vi "cRIO HOST.vi"(8 "error in":errorcluster, 10 "resource name":T1 caption="RIO Device", 11 "MeasSet":T2={"Data Rate 9775"=20.0, "Data Rate 9215"=20.0, "Samples RMS 9215"=10000, "Samples RMS 9775"=10000}) -> (0 "Host error out":errorcluster, 1 "Start time":timestamp=timestamp(3682932872.9709415 s since 1904-01-01), 2 "data 9775x2":dbl[](array[numeric])=[-0.002410888671875, 3.0517578125e-05, -10.432037353515625, -10.390777587890625, -0.002410888671875, 3.0517578125e-05, -10.432037353515625, -10.390777587890625, -0.002105712890625, 0.00067138671875, -10.432037353515625, -10.390777587890625, -0.002410888671875, -0.000274658203125, -10.432037353515625, -10.390777587890625, -0.002105712890625, 3.0517578125e-05, -10.432037353515625, -10.390777587890625, -0.002410888671875, 3.0517578125e-05, -10.432037353515625, -10.390777587890625, -0.002410888671875, 0.0003662109375, -10.432037353515625, -10.390777587890625, -0.002105712890625, -0.000274658203125, -10.432037353515625, -10.390777587890625, -0.0030517578125, 0.00067138671875, -10.432037353515625, -10.390777587890625, -0.0030517578125, -0.000274658203125, -10.432037353515625, -10.390777587890625, -0.002410888671875, 3.0517578125e-05, -10.432037353515625, -10.390777587890625, -0.00274658203125, -0.000274658203125, -10.432037353515625, -10.390777587890625, -0.0030517578125, -0.000274658203125, -10.432037353515625, -10.390777587890625, -0.002410888671875, 0.0003662109375, -10.432037353515625, -10.390777587890625, -0.003387451171875, 3.0517578125e-05, -10.432037353515625, -10.390777587890625, -0.00274658203125, -0.000274658203125, -10.432037353515625, -10.390777587890625, -0.00274658203125, 3.0517578125e-05, -10.432037353515625, -10.390777587890625, -0.002410888671875, -0.000274658203125, -10.432037353515625, -10.390777587890625, -0.002410888671875, 0.0003662109375, -10.432037353515625, -10.390777587890625, -0.00274658203125, 0.0003662109375, -10.432037353515625, -10.390777587890625, -0.002410888671875, 3.0517578125e-05, -10.432037353515625, -10.390777587890625, -0.002410888671875, 3.0517578125e-05, -10.432037353515625, -10.390777587890625, -0.00274658203125, -0.000274658203125, -10.432037353515625, -10.390777587890625, -0.003692626953125, 3.0517578125e-05, -10.432037353515625, -10.390777587890625, -0.002410888671875, 3.0517578125e-05, -10.432037353515625, -10.390777587890625, -0.0030517578125, 3.0517578125e-05, -10.432037353515625, -10.390777587890625, -0.003387451171875, 0.0003662109375, -10.432037353515625, -10.390777587890625, -0.003387451171875, 0.0003662109375, -10.432037353515625, -10.390777587890625, -0.0030517578125, 0.00067138671875, -10.432037353515625, -10.390777587890625, -0.0030517578125, 3.0517578125e-05, -10.432037353515625, -10.390777587890625, -0.0030517578125, 0.0003662109375, -10.432037353515625, -10.390777587890625, -0.0030517578125, 3.0517578125e-05, -10.432037353515625, -10.390777587890625], 3 "data 9215":dbl[](array[numeric])=[0.00146484375, 0.00048828125, -0.0029296875, 0.001953125, 0.0009765625, 0.002197265625, 0.0048828125, -0.000732421875, -0.002685546875, -0.002197265625, -0.00146484375, 0.004638671875, -0.000244140625, -0.000732421875, 0.002197265625, -0.000732421875, -0.002685546875, -0.0009765625, 0.001220703125, -0.0009765625, 0.00244140625, -0.006103515625, 0.0048828125, 0.001953125, 0.0, -0.002197265625, 0.0, 0.001953125, 0.003662109375, -0.00341796875, 0.010498046875, -0.000732421875, -0.002685546875, -0.005126953125, 0.0, 0.003173828125, -0.001708984375, 0.000732421875, 0.002197265625, -0.000732421875, -0.004150390625, -0.002197265625, -0.0068359375, 0.003173828125, 0.00244140625, -0.000732421875, 0.00341796875, 0.00341796875, 0.007080078125, -0.0009765625, 0.001220703125, 0.00048828125, -0.00439453125, -0.000732421875, 0.002197265625, 0.00341796875, 0.0, -0.002197265625, -0.00146484375, 0.003173828125, -0.00439453125, -0.00341796875, 0.000732421875, 0.001953125, -0.002685546875, -0.002197265625, 0.0068359375, 0.001953125, -0.003173828125, -0.000732421875, 0.002197265625, 0.001953125, 0.0029296875, 0.00048828125, 0.002685546875, -0.0009765625, -0.001708984375, -0.000732421875, 0.002197265625, -0.000732421875, 0.0, -0.002197265625, 0.002685546875, -0.002197265625, -0.000244140625, 0.000732421875, 0.007568359375, 0.001953125, -0.00537109375, -0.0009765625, -0.0029296875, 0.001953125, 0.0009765625, 0.002197265625, 0.00634765625, 0.00341796875, -0.001220703125, 0.001953125, -0.00146484375, 0.00048828125, -0.000244140625, -0.004638671875, 0.00341796875, 0.0048828125, 0.0, -0.003662109375, 0.0, 0.001953125, 0.00244140625, 0.000732421875, 0.0048828125, 0.001953125, 0.00146484375, -0.002197265625, 0.002685546875, -0.002197265625, -0.000244140625, 0.000732421875, 0.00341796875, 0.000732421875, 0.00146484375, 0.001953125, -0.00146484375, 0.003173828125, -0.000244140625, -0.000732421875, 0.0048828125, 0.000732421875, 0.00146484375, -0.003662109375, 0.001220703125, 0.00048828125, -0.003173828125, -0.001953125, 0.00634765625, -0.002197265625, 0.004150390625, -0.002197265625, 0.002685546875, 0.001953125, -0.005859375, -0.000732421875, 0.0048828125, 0.00341796875, 0.00146484375, 0.00048828125, 0.0, 0.003173828125, 0.0009765625, 0.000732421875, 0.007568359375, 0.006103515625, -0.001220703125, -0.0009765625, 0.002685546875, 0.001953125, -0.00439453125, -0.00341796875, 0.007568359375, 0.001953125, 0.004150390625, -0.0078125, -0.00146484375, 0.00048828125, -0.00439453125, -0.004638671875, 0.0048828125, 0.00341796875, 0.0, -0.002197265625, -0.00146484375, 0.003173828125, -0.00439453125, -0.000732421875, 0.00634765625, 0.001953125, 0.0, -0.003662109375, 0.0, 0.004638671875, -0.000244140625, -0.004638671875, 0.009033203125, 0.000732421875, -0.002685546875, -0.005126953125, 0.0, 0.00048828125, -0.005859375, -0.001953125, 0.00341796875, -0.00341796875, 0.004150390625, -0.003662109375, 0.004150390625, -0.002197265625, -0.000244140625, -0.00341796875, 0.00341796875, -0.00341796875, 0.004150390625, -0.002197265625, -0.0029296875, -0.002197265625, 0.00244140625, -0.000732421875, 0.0048828125, -0.000732421875, 0.0029296875, 0.00048828125, 0.004150390625, 0.00048828125, 0.00244140625, 0.000732421875, 0.002197265625, -0.00341796875, -0.001220703125, 0.00048828125, 0.0, -0.0009765625, -0.001708984375, -0.000732421875, 0.0048828125, 0.000732421875, -0.001220703125, -0.0009765625, 0.0, 0.006103515625, -0.003173828125, -0.00341796875, 0.0048828125, 0.006103515625, -0.002685546875, -0.00634765625, 0.001220703125, -0.002197265625, -0.00439453125, 0.000732421875, 0.002197265625, 0.000732421875, 0.0, 0.00048828125, -0.00146484375, -0.003662109375, -0.000244140625, -0.000732421875, -0.000732421875, -0.002197265625, -0.001220703125, -0.0009765625, 0.0, -0.003662109375, -0.000244140625, 0.000732421875, -0.000732421875, 0.001953125, -0.001220703125, -0.002197265625, 0.0, 0.003173828125, 0.0009765625, -0.000732421875, -0.000732421875, 0.000732421875, -0.002685546875, -0.002197265625, 0.0, 0.00048828125, -0.001708984375, 0.002197265625, 0.00341796875, -0.0048828125, 0.0, -0.002197265625, 0.001220703125, 0.00048828125, -0.005859375, 0.000732421875, 0.0048828125, 0.001953125, -0.001220703125, -0.003662109375, 0.001220703125, 0.00048828125, -0.00439453125, 0.000732421875, 0.0048828125, -0.002197265625, -0.001220703125, 0.001953125, 0.004150390625, 0.001953125, -0.001708984375, 0.000732421875, 0.00634765625, 0.0048828125, -0.004150390625, -0.0009765625, 0.001220703125, -0.0009765625, 0.0009765625, -0.001953125, 0.002197265625, -0.002197265625, -0.002685546875, -0.002197265625, 0.0, 0.00732421875, 0.0009765625, -0.001953125, 0.0048828125, 0.000732421875, 0.00146484375, -0.003662109375, 0.002685546875, 0.003173828125, -0.00439453125, -0.004638671875, -0.001953125, 0.001953125, -0.004150390625, -0.005126953125, 0.004150390625, 0.00048828125, 0.003662109375, -0.00341796875, -0.001953125, 0.0048828125, -0.002685546875, -0.0009765625, 0.0, 0.003173828125, 0.0009765625, -0.000732421875, 0.00634765625, -0.000732421875, 0.00146484375, 0.001953125, 0.001220703125, 0.00048828125, 0.0009765625, -0.000732421875, 0.002197265625, 0.00341796875, -0.001220703125, -0.002197265625, 0.0, 0.00048828125, 0.0009765625, -0.001953125, 0.002197265625, -0.000732421875, 0.00146484375, -0.0009765625, 0.002685546875, 0.003173828125, 0.00244140625, -0.000732421875, 0.00634765625, 0.001953125, 0.0, -0.002197265625, -0.0029296875, 0.003173828125, -0.000244140625, -0.001953125, -0.001953125, 0.001953125, -0.001220703125, 0.003173828125, -0.0029296875, 0.003173828125, -0.00439453125, -0.001953125, 0.00634765625, -0.002197265625, -0.001220703125, 0.001953125, -0.0029296875, 0.00048828125, 0.003662109375, 0.000732421875, 0.002197265625, 0.001953125, 0.0, -0.0009765625, -0.00146484375, 0.003173828125, -0.00439453125, -0.001953125, 0.0048828125, 0.000732421875, 0.00146484375, -0.0009765625, 0.002685546875, 0.00048828125, 0.003662109375, -0.000732421875, -0.000732421875, -0.000732421875, 0.0, 0.003173828125, -0.004150390625, 0.003173828125, 0.0009765625, 0.0048828125, 0.00341796875, 0.0048828125, -0.004150390625, 0.001953125, 0.002685546875, 0.001953125, 0.003662109375, 0.002197265625, 0.00634765625, -0.000732421875, -0.001220703125, 0.001953125, 0.002685546875, 0.001953125, -0.001708984375, 0.00341796875, 0.009033203125, 0.000732421875, -0.001220703125, -0.002197265625, 0.0, 0.003173828125, 0.003662109375, 0.000732421875, 0.009033203125, -0.00634765625, 0.0029296875, -0.0009765625, -0.00146484375, -0.002197265625, 0.0009765625, -0.000732421875, 0.00634765625, 0.000732421875, -0.004150390625, -0.005126953125, 0.001220703125, 0.00048828125, 0.0009765625, 0.00341796875, 0.009033203125, -0.002197265625, 0.00146484375, 0.00048828125, 0.0, 0.003173828125, -0.000244140625, -0.004638671875, 0.0048828125, 0.000732421875, -0.00537109375, -0.002197265625, -0.004150390625, -0.0009765625, -0.001708984375, -0.000732421875, 0.00634765625, -0.002197265625, 0.0029296875, 0.00048828125, -0.0029296875, 0.00048828125, -0.000244140625, 0.000732421875, 0.00634765625, 0.0048828125, -0.001220703125, -0.003662109375, 0.001220703125, -0.002197265625, -0.005859375, -0.00341796875, 0.00341796875, 0.001953125, -0.002685546875, -0.0009765625, 0.0, -0.002197265625, -0.005859375, -0.000732421875, 0.00634765625, 0.001953125, 0.004150390625, -0.003662109375, 0.001220703125, 0.00048828125, -0.001708984375, 0.000732421875, 0.002197265625, 0.000732421875, 0.00146484375, -0.003662109375, -0.00146484375, -0.002197265625, -0.003173828125, -0.00341796875, 0.00341796875, 0.00341796875, 0.0, 0.001953125, 0.004150390625, 0.006103515625, -0.001708984375, 0.00341796875, 0.002197265625, -0.000732421875, 0.004150390625, -0.0009765625, 0.008056640625, 0.003173828125, -0.000244140625, -0.001953125, 0.007568359375, 0.00341796875, -0.004150390625, 0.003173828125, 0.002685546875, 0.003173828125, -0.001708984375, -0.000732421875, 0.0048828125, 0.001953125, -0.00537109375, -0.002197265625, -0.00146484375, -0.002197265625, 0.00244140625, -0.000732421875, 0.0048828125, 0.001953125, 0.00146484375, -0.0009765625, 0.004150390625, 0.003173828125, 0.0009765625, -0.004638671875, 0.000732421875, 0.001953125, 0.0, 0.001953125, 0.002685546875, 0.001953125, -0.000244140625, -0.00341796875, 0.0048828125, 0.000732421875, -0.001220703125, 0.003173828125, 0.0, 0.00048828125, -0.000244140625, 0.000732421875, 0.0048828125, 0.00341796875, 0.00146484375, 0.001953125, 0.002685546875, -0.0009765625, -0.000244140625, 0.000732421875, 0.002197265625, 0.00341796875, -0.001220703125, -0.003662109375, 0.001220703125, 0.00048828125, -0.000244140625, 0.000732421875, 0.00341796875, 0.00341796875, 0.0, -0.005126953125, 0.002685546875, 0.003173828125, -0.003173828125, 0.0048828125, 0.0048828125, 0.001953125, 0.0, -0.0009765625, 0.002685546875, 0.001953125, -0.00439453125, -0.000732421875, 0.00341796875, 0.0048828125, -0.001220703125, -0.0009765625, 0.004150390625, 0.001953125, -0.005859375, 0.000732421875, 0.0048828125, 0.000732421875, 0.007080078125, -0.002197265625, 0.004150390625, 0.001953125, -0.000244140625, -0.000732421875, 0.00341796875, 0.001953125, -0.002685546875, 0.003173828125, -0.0029296875, -0.002197265625, -0.001708984375, -0.004638671875, 0.00634765625, 0.001953125, -0.004150390625, -0.0009765625, 0.001220703125, 0.001953125, -0.00439453125, 0.00341796875, 0.00341796875, 0.00341796875, 0.00146484375, 0.003173828125, 0.0, 0.003173828125, -0.000244140625, -0.000732421875, 0.00634765625, -0.002197265625, 0.0, 0.001953125, 0.001220703125, 0.001953125, -0.00439453125, 0.00341796875, 0.000732421875, 0.001953125, 0.00146484375, 0.00048828125, 0.001220703125, 0.003173828125, -0.00732421875, 0.000732421875, 0.002197265625, -0.000732421875, -0.004150390625, 0.003173828125, -0.00146484375, 0.003173828125, -0.000244140625, -0.001953125, 0.00341796875, -0.000732421875, 0.007080078125, 0.003173828125, 0.004150390625, -0.002197265625, 0.0009765625, -0.000732421875, 0.0048828125, 0.001953125, -0.001220703125, -0.0009765625, -0.00146484375, 0.001953125, -0.00732421875, -0.000732421875, 0.0048828125, -0.000732421875, -0.004150390625, 0.001953125, 0.001220703125, 0.003173828125, -0.00732421875, 0.000732421875, 0.007568359375, -0.00341796875, 0.00146484375, -0.002197265625, 0.004150390625, -0.0009765625, -0.00439453125, -0.001953125, 0.0048828125, 0.000732421875, -0.00537109375, 0.00048828125, 0.001220703125, 0.00048828125, -0.00439453125, -0.00341796875, 0.0048828125, -0.000732421875, -0.002685546875, 0.00048828125, 0.0, 0.001953125, -0.001708984375, -0.000732421875, 0.0048828125, -0.000732421875, 0.0, -0.002197265625, 0.001220703125, -0.0009765625, -0.005859375, -0.000732421875, 0.000732421875, 0.00341796875, -0.002685546875, -0.0009765625, 0.0, -0.0009765625, 0.0009765625, -0.00341796875, 0.00634765625, 0.00341796875, -0.002685546875, -0.002197265625, 0.002685546875, 0.001953125, 0.0009765625, -0.001953125, 0.000732421875, -0.002197265625, 0.0029296875, 0.00048828125, -0.00146484375, 0.001953125, -0.00439453125, -0.00341796875, 0.007568359375, -0.000732421875, 0.0029296875, 0.001953125, 0.004150390625, 0.003173828125, -0.000244140625, -0.001953125, 0.00341796875, 0.000732421875, -0.00537109375, 0.00048828125, 0.0, 0.00048828125, -0.000244140625, -0.00341796875, -0.001953125, -0.002197265625, 0.0, -0.003662109375, -0.00146484375, -0.0009765625, -0.003173828125, -0.001953125, 0.0048828125, 0.000732421875, 0.00146484375, 0.00048828125, 0.0, 0.00048828125, 0.00244140625, -0.000732421875, 0.00341796875, 0.000732421875, -0.00537109375, -0.002197265625, -0.0029296875, 0.001953125, -0.003173828125, -0.000732421875, 0.0048828125, 0.000732421875, -0.002685546875, -0.002197265625, 0.001220703125, -0.002197265625, -0.000244140625, -0.001953125, 0.0048828125, -0.000732421875, -0.002685546875, 0.001953125, 0.0, 0.001953125, -0.000244140625, -0.001953125, 0.009033203125, 0.000732421875, -0.001220703125, 0.003173828125, 0.001220703125, -0.0009765625, -0.00732421875, -0.006103515625, 0.000732421875, -0.002197265625, -0.00537109375, -0.002197265625, -0.00146484375, -0.002197265625, -0.000244140625, -0.0087890625, 0.00341796875, 0.000732421875, -0.001220703125, 0.00048828125, 0.001220703125, -0.003662109375, -0.000244140625, -0.000732421875, 0.00341796875, 0.001953125, -0.002685546875, 0.003173828125, -0.004150390625, -0.0009765625, -0.001708984375, 0.00341796875, 0.000732421875, -0.000732421875, -0.002685546875, -0.0009765625, 0.002685546875, -0.002197265625, -0.001708984375, -0.001953125, 0.00341796875, 0.000732421875, -0.004150390625, -0.0009765625, -0.00146484375, -0.002197265625, 0.003662109375, -0.001953125, 0.0048828125, -0.00341796875, 0.00146484375, -0.003662109375, -0.00146484375, 0.00048828125, -0.000244140625, -0.000732421875, 0.007568359375, 0.00341796875, 0.0029296875, 0.001953125, -0.004150390625, -0.0009765625, -0.00439453125, 0.0048828125, 0.00341796875, -0.00341796875, -0.002685546875, 0.004638671875, 0.001220703125, 0.001953125, -0.003173828125, -0.000732421875, -0.000732421875, -0.00634765625, -0.004150390625, 0.001953125, 0.0, 0.003173828125, -0.000244140625, -0.000732421875, 0.000732421875, 0.001953125, 0.00146484375, -0.002197265625, 0.001220703125, 0.001953125, 0.0009765625, -0.001953125, 0.0048828125, -0.000732421875, -0.004150390625, -0.002197265625, 0.002685546875, -0.0009765625, -0.001708984375, 0.000732421875, 0.00341796875, 0.001953125, 0.00146484375, 0.001953125, 0.004150390625, -0.0009765625, 0.0009765625, -0.00341796875, 0.00341796875, -0.002197265625], 4 "Data FIFO Full":bool=TRUE, 6 "Data2 FIFO Full":bool=TRUE)   [LabVIEW 2019, in "DAQ_Engine.lvclass"]
uses:
  DAQ_Engine.lvclass
  Common/DataTypes/Measurement Config--cluster.ctl
  <vilib>/userdefined/High Color/nirio_resource_hc.ctl
  <vilib>/LabVIEW Targets/FPGA/cRIO/shared/nicrio_ModuleControls/nicrio_BasicConversionTime.ctl
  <vilib>/rvi/interface/RandomDataEmulation/nirviRandomDataOpen.vi
  <vilib>/rvi/interface/common/niFpgaCacheSessionInfoDynamic.vi
  <vilib>/Utility/error.llb/Error Cluster From Error Code.vi
  <vilib>/rvi/errors/niLvFpgaAdjustHostInterfaceError.vi
  <vilib>/FPGAPlugInAG/Dynamic/niLvFpga_Run_Dynamic.vi
  <vilib>/FPGAPlugInAG/Dynamic/niLvFpga_Close_Dynamic.vi
  <vilib>/rvi/interface/nirviOpenFPGA/nirviOpenFPGA.xnode
  FPGA/Acquisitions (FPGA).vi
  <vilib>/rvi/interface/nirviReadWriteControl/nirviReadWriteControl.xnode
  <vilib>/rvi/interface/nirviMethod/nirviMethod.xnode
  <vilib>/rvi/interface/nirviCloseFPGA/nirviCloseFPGA.xnode
  <vilib>/FPGAPlugInAG/Dynamic/niLvFpga_ReadFifo_Dynamic.vi
  <vilib>/rvi/errors/niLvFpgaMergeErrorWithErrorCode.vi
  <vilib>/rvi/interface/Simulation/niFpgaSimulationCallBeginRW.vi
  NiFpgaLv.dll
panel:
  out "Elements Remaining 2":u32=15488
  in  "stop":bool
  out "FPGA error out":errorcluster
  out "Elements Remaining":u32=3967
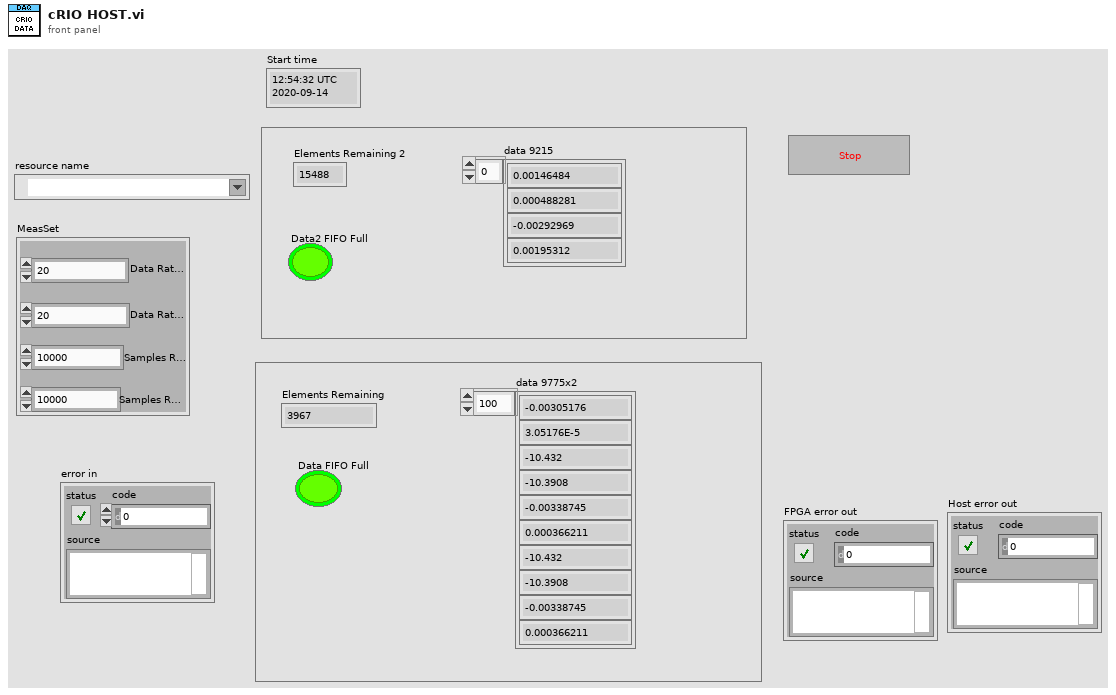
[diagram p1: front panel]
types:
  T1 = typedef "nirio_resource_hc.ctl" = tag
  T2 = typedef "Measurement Config--cluster.ctl" = cluster{"Data Rate 9775":dbl, "Data Rate 9215":dbl, "Samples RMS 9215":u32, "Samples RMS 9775":u32}
  T3 = typedef "nicrio_BasicConversionTime.ctl" = enum8{"High Speed", "High Resolution"}
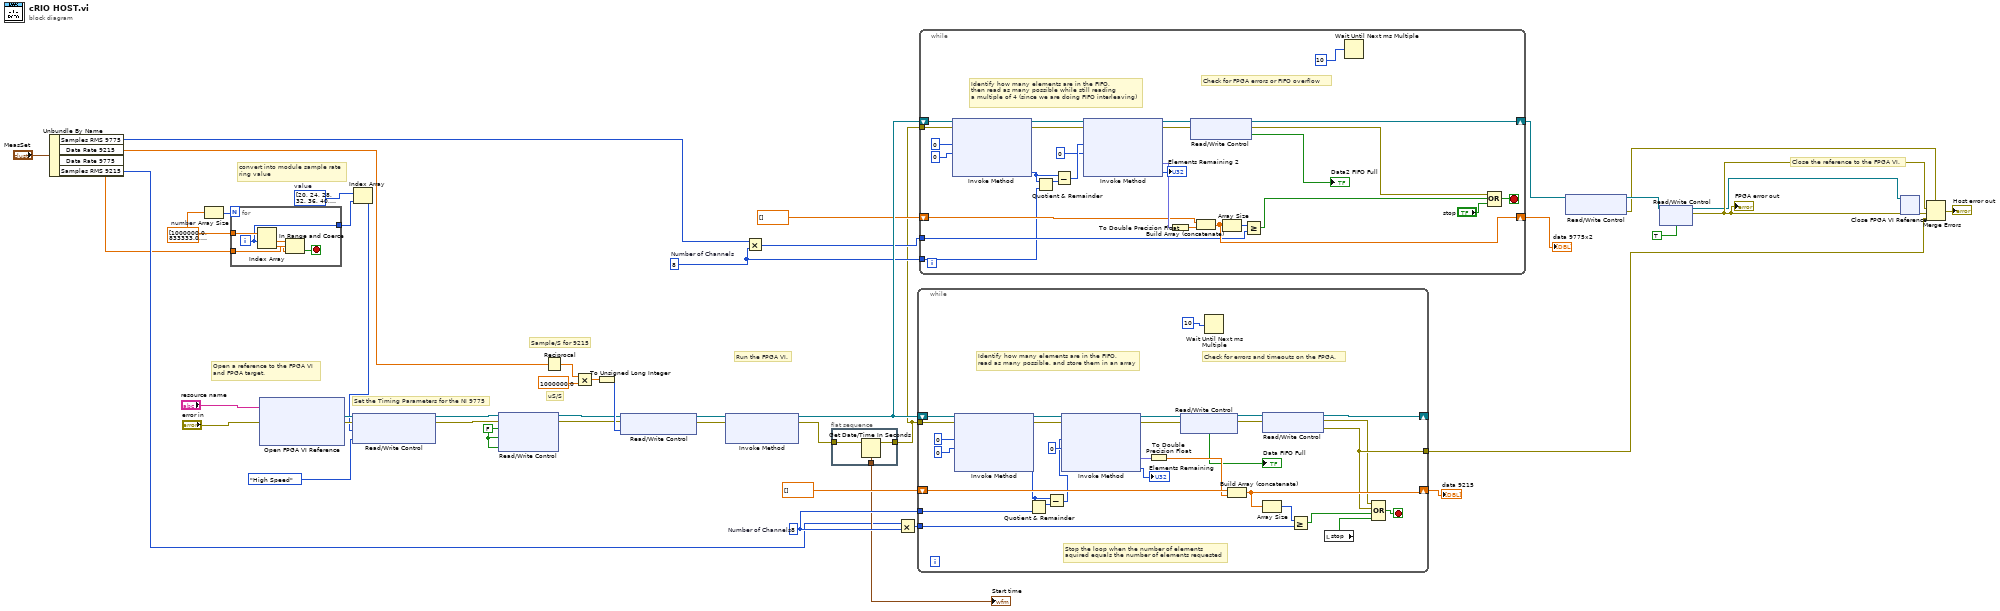
[diagram p0: block diagram]
diagram:
  w3 = u16[] [20, 24, 28, 32, 36, 40, 44, 48, 52, 56, 60, 64, 68, 72, 76, 80, 84, 88, 92, 96, 100, 104, 108, 112, 116, 120, 124, 128, 132, 136, 140, 144, 148, 152, 156, 160, 164, 168, 172, 176, 180, 184, 188, 192, 196, 200, 400, 600, 800, 1000, 1200, 1400, 1600, 1800, 2000, 2200, 2400, 2600, 2800, 3000, 3200, 3400, 3600, 4000, 4200, 4400, 4600, 4800, 5000, 5200, 5600, 6000, 6400, 6800, 7200, 7600, 8000, 8400, 8800, 9200, 9600, 10000, 10400, 10800, 11200, 11600, 12000, 12400, 12800, 13200, 13600, 14000, 14400, 14800, 15200, 15600, 16000, 16400, 16800, 17200, 17600, 18000, 18400, 18800, 19200, 19600, 20000, 20400, 20800, 21200, 21600, 22000, 22400, 22800, 23200, 23600, 24000, 24400, 24800, 25200, 25600, 28800, 32000, 35200, 38400, 44800, 51200, 57600, 64000]  # value
  w5 = dbl[] [1000000.0, 833333.0, 714286.0, 625000.0, 555556.0, 500000.0, 454545.0, 416667.0, 384615.0, 357143.0, 333333.0, 312500.0, 294118.0, 277778.0, 263158.0, 250000.0, 238095.0, 227273.0, 217391.0, 208333.0, 200000.0, 192308.0, 185185.0, 178571.0, 172414.0, 166667.0, 161290.0, 156250.0, 151515.0, 147059.0, 142857.0, 138889.0, 135135.0, 131579.0, 128205.0, 125000.0, 121951.0, 119048.0, 116279.0, 113636.0, 111111.0, 108696.0, 106383.0, 104167.0, 102041.0, 100000.0, 50000.0, 33333.0, 25000.0, 20000.0, 16667.0, 14286.0, 12500.0, 11111.0, 10000.0, 9091.0, 8333.0, 7692.0, 7143.0, 6667.0, 6250.0, 5882.0, 5556.0, 5000.0, 4762.0, 4545.0, 4348.0, 4167.0, 4000.0, 3846.0, 3571.0, 3333.0, 3125.0, 2941.0, 2778.0, 2632.0, 2500.0, 2381.0, 2273.0, 2174.0, 2083.0, 2000.0, 1923.0, 1852.0, 1786.0, 1724.0, 1667.0, 1613.0, 1563.0, 1515.0, 1471.0, 1429.0, 1389.0, 1351.0, 1316.0, 1282.0, 1250.0, 1220.0, 1190.0, 1163.0, 1136.0, 1111.0, 1087.0, 1064.0, 1042.0, 1020.0, 1000.0, 980.0, 962.0, 943.0, 926.0, 909.0, 893.0, 877.0, 862.0, 847.0, 833.0, 820.0, 806.0, 794.0, 781.0, 694.0, 625.0, 568.0, 521.0, 446.0, 391.0, 347.0, 313.0]  # number
  w18 = FALSE ("Data2 FIFO Full")
  w32 = u32 8  # Number of Channels
  w35 = u32 8  # Number of Channels
  # "convert into module sample rate\nring value"
  # "Sample/S for 9215"
  # "uS/S"
  # "Set the Timing Parameters for the NI 9775"
  # "Close the reference to the FPGA VI."
  # "Run the FPGA VI."
  # "Open a reference to the FPGA VI \nand FPGA target."
  n1 = Unbundle By Name("MeasSet") -> ("Samples RMS 9775"=w25:u32, "Data Rate 9215"=w11:dbl, "Data Rate 9775"=w6:dbl, "Samples RMS 9215"=w24:u32)
  n2 = Array Size(array=w5) -> (size(s)=w4:i32)
  n3 = for {
    N: w4 -> [_]
    tunnel: w5 -> [w53]
    tunnel: w6 -> [w51]
    tunnel: [w48] -> w2
    i -> [w48]
    stop <- w49 stop-if-true
    n4 = Index Array(array=w53, index #1=w48) -> (element #1=w52:dbl, element #2=w50:dbl)  [unwired: 1 in]
    n5 = In Range and Coerce(upper limit=w52, x=w51, lower limit=w50) -> (In Range?=w49:bool)  [unwired: 1 out]
  }
  n6 = xnode "Open FPGA VI Reference"("error in"="error in", "resource name"="resource name") -> ("FPGA VI Reference Out"=w39:refnum<k20>, "error out"=w44:errorcluster)
  n7 = Index Array(array=w3, index=w2) -> (element=w1:u16)
  n8 = xnode "Read/Write Control"("FPGA VI Reference In"=w39, "error in"=w44, "Continuous Data Rate"=w1, "Timing Mode"=nicrio_BasicConversionTime."High Speed") -> ("FPGA VI Reference Out"=w23:refnum<k20>, "error out"=w21:errorcluster)
  n9 = xnode "Read/Write Control"("FPGA VI Reference In"=w23, "error in"=w21, "Data2 FIFO Full"=w18, "Data FIFO Full"=w18, "Stop"=w18) -> ("FPGA VI Reference Out"=w22:refnum<k20>, "error out"=w20:errorcluster)
  n10 = Reciprocal(x=w11) -> (1/x=w43:dbl)
  n11 = Multiply(x=w43, y=1000000.0) -> (x*y=w41:dbl)
  n12 = To Unsigned Long Integer(number=w41) -> (unsigned 32bit integer=w40:u32)
  n13 = xnode "Read/Write Control"("FPGA VI Reference In"=w22, "error in"=w20, "Loop Rate 9215 (uS)"=w40) -> ("FPGA VI Reference Out"=w37:refnum<k20>, "error out"=w38:errorcluster)
  n14 = xnode "Invoke Method"("FPGA VI Reference In"=w37, "error in"=w38) -> ("FPGA VI Reference Out"=w36:refnum<k20>, "error out"=w29:errorcluster)  [unwired: 1 in]
  n15 = Multiply(x=w25, y=w32) -> (x*y=w33:u32)
  n16 = flat-sequence {
    tunnel: w29 -> [w55]
    tunnel: [w55] -> w28
    tunnel: [w54] -> w27
    frame #0 {
      n17 = Get Date/Time In Seconds() -> (seconds since 1Jan1904=w54:timestamp)
    }
  }
  n18 = Multiply(x=w24, y=w35) -> (x*y=w46:u32)
  n19 = while {
    shift-right: [w61] -> _
    shift-left: w36 -> [w80]
    shift-right: [w74] -> w8
    shift-left: dbl[] [] -> [w76]
    tunnel: w46 -> [w72]
    tunnel: w28 -> [w79]
    tunnel: [w70] -> w10
    tunnel: w35 -> [w65]
    stop <- w59 stop-if-true
    # "Check for errors and timeouts on the FPGA."
    # "Stop the loop when the number of elements\naquired equals the number of elements requested"
    # "Identify how many elements are in the FIFO, \nread as many possible, and store them in an array"
    n20 = xnode "Invoke Method"("FPGA VI Reference In"=w80, "error in"=w79, "Number of Elements"=u32 0, "Timeout (ms)"=0) -> ("FPGA VI Reference Out"=w78:refnum<k20>, "error out"=w77:errorcluster, "Elements Remaining"=w67:u32)  [unwired: 1 out]
    n21 = Quotient & Remainder(x=w67, y=w65) -> (x-y*floor(x/y)=w68:u32)  [unwired: 1 out]
    n22 = Subtract(x=w67, y=w68) -> (x-y=w66:u32)
    n23 = xnode "Invoke Method"("FPGA VI Reference In"=w78, "error in"=w77, "Number of Elements"=w66, "Timeout (ms)"=0 ("Timeout")) -> ("FPGA VI Reference Out"=w62:refnum<k20>, "error out"=w64:errorcluster, "Data"=w83:fxp<+/-,20,5>[], "Elements Remaining"=→"Elements Remaining":u32)
    n24 = To Double Precision Float(number=w83) -> (double precision float=w75:dbl[])
    n25 = xnode "Read/Write Control"("FPGA VI Reference In"=w62, "error in"=w64) -> ("FPGA VI Reference Out"=w63:refnum<k20>, "error out"=w60:errorcluster, "Data FIFO Full"=→"Data FIFO Full":bool)
    n26 = Wait Until Next ms Multiple(millisecond multiple=u32 10 ("Host Loop update rate 9775 (ms)")) -> ()  [unwired: 1 out]
    n27 = Build Array (concatenate)(w76, w75) -> (w74:dbl[])
    n28 = xnode "Read/Write Control"("FPGA VI Reference In"=w63, "error in"=w60) -> ("FPGA VI Reference Out"=w61:refnum<k20>, "error out"=w56:errorcluster, "FPGA Error Out"=w70:errorcluster)
    n29 = Array Size(array=w74) -> (size(s)=w73:i32)
    n30 = Greater Or Equal?(x=w73, y=w72) -> (x >= y?=w71:bool)
    n31 = local read "stop"() -> (w69:bool)
    n32 = Compound Arithmetic op=OR(w56, w70, w71, w69) -> (w59:bool)
  }
  "data 9215" <- w8
  n33 = while {
    tunnel: w28 -> [w103]
    tunnel: w33 -> [w90]
    shift-right: [w92] -> w7
    shift-left: dbl[] [] -> [w95]
    tunnel: w32 -> [w88]
    shift-right: [w86] -> w15
    shift-left: w36 -> [w104]
    stop <- w100 stop-if-true
    # "Check for FPGA errors or FIFO overflow"
    # "Identify how many elements are in the FIFO, \nthen read as many possible while still reading\na multiple of 4 (since we are doing FIFO interleaving)"
    n34 = xnode "Invoke Method"("FPGA VI Reference In"=w104, "error in"=w103, "Number of Elements"=u32 0, "Timeout (ms)"=0) -> ("FPGA VI Reference Out"=w110:refnum<k20>, "error out"=w105:errorcluster, "Elements Remaining"=w108:u32)  [unwired: 1 out]
    n35 = Quotient & Remainder(x=w108, y=w88) -> (x-y*floor(x/y)=w109:u32)  [unwired: 1 out]
    n36 = Subtract(x=w108, y=w109) -> (x-y=w107:u32)
    n37 = xnode "Invoke Method"("FPGA VI Reference In"=w110, "error in"=w105, "Number of Elements"=w107, "Timeout (ms)"=0) -> ("FPGA VI Reference Out"=w102:refnum<k20>, "error out"=w101:errorcluster, "Data"=w96:fxp<+/-,17,5>[], "Elements Remaining"=→"Elements Remaining 2":u32)
    n38 = To Double Precision Float(number=w96) -> (double precision float=w94:dbl[])
    n39 = xnode "Read/Write Control"("FPGA VI Reference In"=w102, "error in"=w101) -> ("FPGA VI Reference Out"=w86:refnum<k20>, "error out"=w97:errorcluster, "Data2 FIFO Full"=→"Data2 FIFO Full":bool)
    n40 = Build Array (concatenate)(w95, w94) -> (w92:dbl[])
    n41 = Array Size(array=w92) -> (size(s)=w93:i32)
    n42 = Greater Or Equal?(x=w93, y=w90) -> (x >= y?=w89:bool)
    n43 = Wait Until Next ms Multiple(millisecond multiple=u32 10 ("Host Loop update rate 9215 (ms)")) -> ()  [unwired: 1 out]
    n44 = Compound Arithmetic op=OR(w97, w89, "stop") -> (w100:bool)
  }
  "data 9775x2" <- w7
  n45 = xnode "Read/Write Control"("FPGA VI Reference In"=w15) -> ("FPGA VI Reference Out"=w14:refnum<k20>, "FPGA Error Out"=w9:errorcluster)  [unwired: 1 in, 1 out]
  n46 = xnode "Read/Write Control"("FPGA VI Reference In"=w14, "Stop"=TRUE) -> ("FPGA VI Reference Out"=w16:refnum<k20>, "error out"=w17:errorcluster)  [unwired: 1 in]
  "FPGA error out" <- w17
  n47 = xnode "Close FPGA VI Reference"("FPGA VI Reference In"=w16, "error in"=w17) -> ("error out"=w47:errorcluster)
  n48 = Merge Errors(w9, w17, w47, w10) -> (→"Host error out":errorcluster)
  "Start time" <- w27
